vi "After Run TS.vi"(8 "error in":errorcluster, 11 "DeepU Test Stand in":refnum<class "DeepU Test Stand.lvclass">) -> (0 "error out":errorcluster, 3 "DeepU Test Stand out":refnum<class "DeepU Test Stand.lvclass">)   [LabVIEW 2019, in "Test Stands.lvlib" / "DeepU Test Stand.lvclass"]
uses:
  DeepU Test Stand.lvclass
  Generic Test Stand/Generic Test Stand.lvclass
  DAC/DAC.lvclass
  C:/Users/krio/Documents/LV_Projects/test-stand/App/Generic Test Stand/Generic Test Stand.lvclass
  DAC/DeepU/HS Vibration/DAC HS Vib.lvclass
  C:/Users/krio/Documents/LV_Projects/test-stand/App/DAC/DAC.lvclass
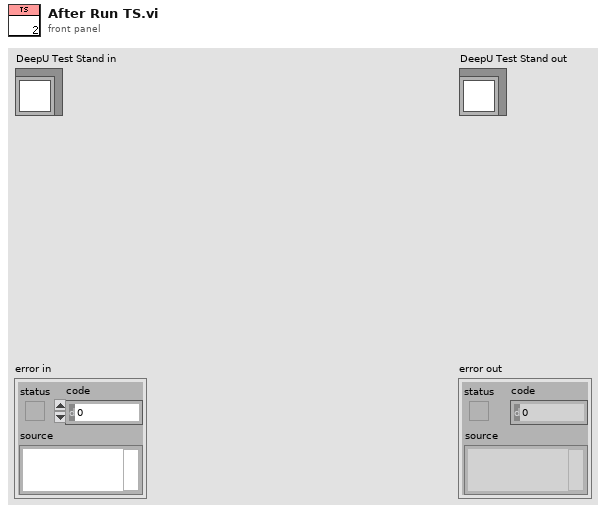
[diagram p1: front panel]
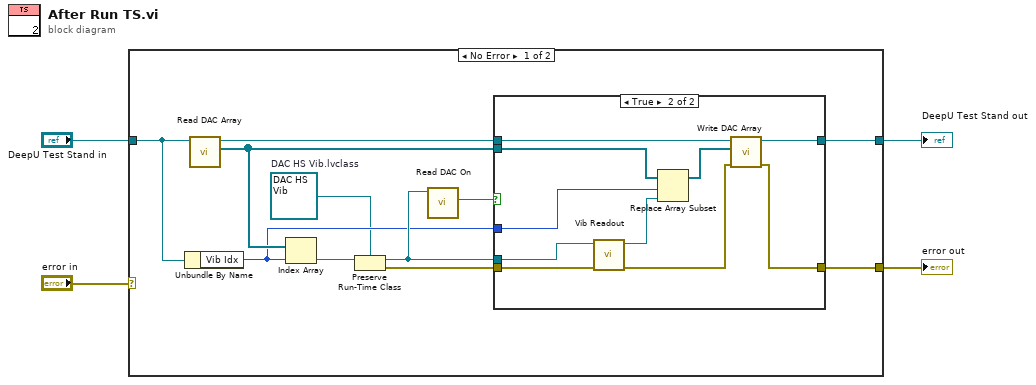
[diagram p0: block diagram]
diagram:
  n1 = case shown="No Error" "error in" {
    selector: "error in" -> [_ w29]
    tunnel: [w6 w29] -> w1
    tunnel: [w7 w28] -> w2
    tunnel: "DeepU Test Stand in" -> [w10 w28]
    frame No Error {
      w5 = refnum<class "DAC HS Vib.lvclass"> refnum  # DAC HS Vib.lvclass
      n2 = Unbundle By Name(w10) -> ("Vib Idx"=w8:i32)
      n3 = call "Read DAC Array.vi"("Generic Test Stand in"=w10) -> ("DAC Array"=w11:refnum<class "DAC.lvclass">[], "Generic Test Stand out"=w14:refnum<class "DeepU Test Stand.lvclass">)  [unwired: 8 in, 1 out]
      n4 = Index Array(array=w11, index=w8) -> (element=w13:refnum<class "DAC.lvclass">)
      n5 = Preserve Run-Time Class(object in=w13, 2:w5) -> (object out=w9:refnum<class "DAC HS Vib.lvclass">, error out=w12:errorcluster)  [unwired: 1 in]
      n6 = call "Read DAC On.vi"("DAC in"=w9) -> ("DAC On"=w15:bool)  [unwired: 8 in, 2 out]
      n7 = case shown="True" w15 {
        tunnel: w14 -> [w17 w25]
        tunnel: [w17 w27] -> w7
        tunnel: w9 -> [_ w20]
        tunnel: w12 -> [w16 w21]
        tunnel: w11 -> [_ w26]
        tunnel: [w16 w23] -> w6
        tunnel: w8 -> [_ w22]
        frame False {
        }
        frame True {
          n8 = call "Vib Readout.vi"("error in"=w21, "DAC HS Vib in"=w20) -> ("error out"=w18:errorcluster, "DAC HS Vib out"=w19:refnum<class "DAC HS Vib.lvclass">)  [unwired: 8 in]
          n9 = Replace Array Subset(array=w26, new element=w19, index=w22) -> (w24:refnum<class "DAC.lvclass">[])
          n10 = call "Write DAC Array.vi"("error in (no error)"=w18, "DAC Array"=w24, "Generic Test Stand in"=w25) -> ("error out"=w23:errorcluster, "Generic Test Stand out"=w27:refnum<class "DeepU Test Stand.lvclass">)  [unwired: 7 in]
        }
      }
    }
    frame Error {
    }
  }
  "error out" <- w1
  "DeepU Test Stand out" <- w2
